vi "Write Range UI.vi"(8 "error in (no error)":errorcluster, 9 "Reader Time":dbl[unit], 10 "Set UI to input? (F)":bool, 11 "Double Scanner in":refnum<class "Double Scanner.lvclass">) -> (0 "error out":errorcluster, 3 "Double Scanner out":refnum<class "Double Scanner.lvclass">)   [LabVIEW 2012, in "Double Scanner.lvclass"]
doc: "A Setup UI method for the superclass \"Range\" of scanner."
uses:
  Double Scanner.lvclass
  Scanner/Scanner.lvclass
  Scanner/Range.ctl
panel:
  out "# Points":u32
  out "Time Estimate":string
  in  "Tab Control":enum32{"Range 1", "Range 2"}(tab)
  in  "First 1":dbl
  in  "Last 1":dbl
  in  "Step Size 1":dbl=1.0 min=0.0
  in  "Return to 1":dbl
  in  "Return to...? 1":bool
  in  "First 2":dbl
  in  "Last 2":dbl
  in  "Step Size 2":dbl=1.0 min=0.0
  in  "Return to 2":dbl
  in  "Return to...? 2":bool
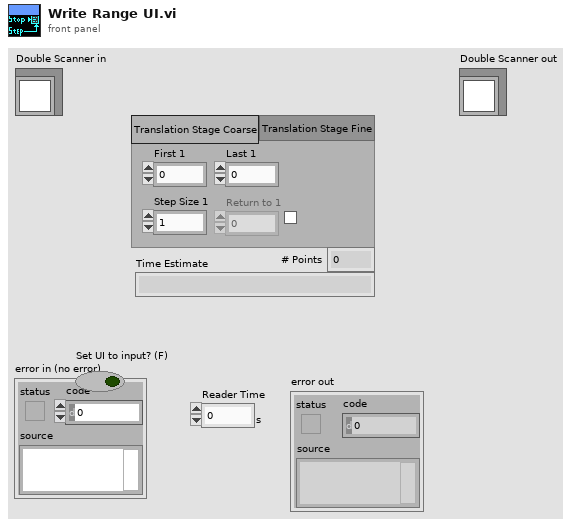
[diagram p1: front panel]
types:
  T1 = typedef "Scanner.lvclass/Range.ctl" = cluster{"xi":dbl, "xf":dbl, "dx":dbl, "Return to...?":bool, "Return to":dbl}
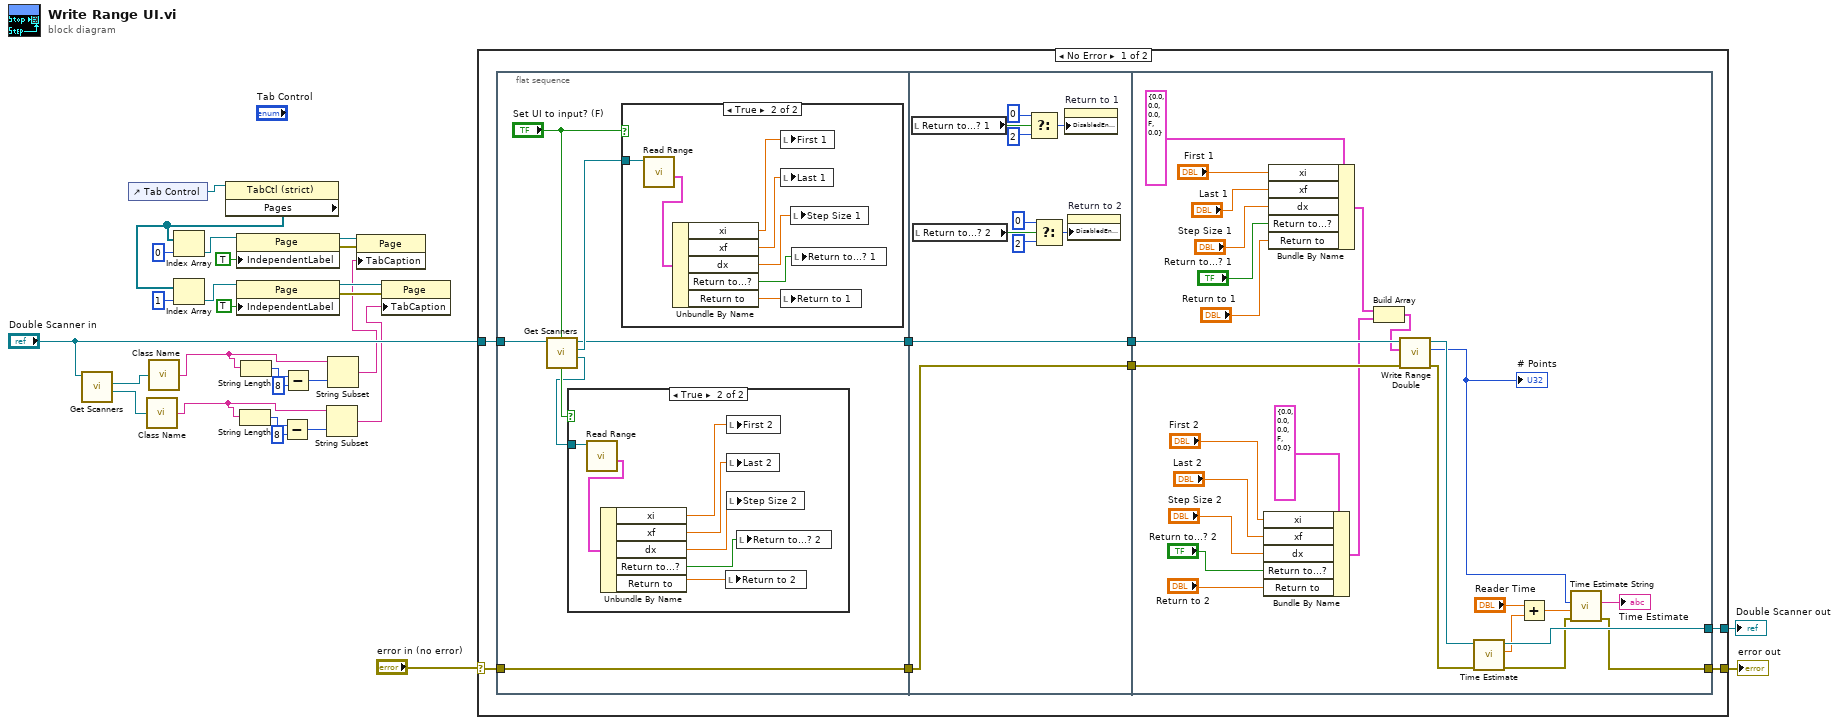
[diagram p0: block diagram]
diagram:
  n1 = call-dynamic "Get Scanners.vi"("Double Scanner in"="Double Scanner in") -> ("Scanner 2 out"=w23:refnum<class "Scanner.lvclass">, "Scanner 1 out"=w24:refnum<class "Scanner.lvclass">)  [unwired: 7 in, 2 out]
  n2 = control-ref of="Tab Control"() -> (w22:refnum<vi>)
  n3 = call "Class Name.vi"("LabVIEW Object"=w23) -> ("Classname"=w1:string)
  n4 = call "Class Name.vi"("LabVIEW Object"=w24) -> ("Classname"=w6:string)
  n5 = property class="TabCtl (strict)"(reference=w22) -> ("Pages"=w20:refnum<vi>[])  [unwired: 1 in, 2 out]
  n6 = Index Array(array=w20, index=0) -> (element=w17:refnum<vi>)
  n7 = Index Array(array=w20, index=1) -> (element=w18:refnum<vi>)
  n8 = property class="Page"(reference=w17, "IndependentLabel"=TRUE ("Independent Label")) -> (reference out=w13:refnum<vi>, error out=w12:errorcluster)  [unwired: 1 in]
  n9 = property class="Page"(reference=w18, "IndependentLabel"=TRUE ("Independent Label")) -> (reference out=w14:refnum<vi>, error out=w11:errorcluster)  [unwired: 1 in]
  n10 = String Length(string=w1) -> (length=w5:i32)
  n11 = String Length(string=w6) -> (length=w10:i32)
  n12 = Subtract(x=w5, y=8) -> (x-y=w3:i32)
  n13 = Subtract(x=w10, y=8) -> (x-y=w7:i32)
  n14 = String Subset(string=w1, length (rest)=w3) -> (substring=w2:string)  [unwired: 1 in]
  n15 = String Subset(string=w6, length (rest)=w7) -> (substring=w8:string)  [unwired: 1 in]
  n16 = property class="Page"(reference=w13, error in=w12, "TabCaption"=w8) -> ()  [unwired: 2 out]
  n17 = property class="Page"(reference=w14, error in=w11, "TabCaption"=w2) -> ()  [unwired: 2 out]
  n18 = case shown="No Error" "error in (no error)" {
    selector: "error in (no error)" -> [w35 w95]
    tunnel: [w33 w95] -> w27
    tunnel: [w34 w94] -> w28
    tunnel: "Double Scanner in" -> [w36 w94]
    frame No Error {
      n19 = flat-sequence {
        tunnel: w35 -> [w42]
        tunnel: w36 -> [w40]
        tunnel: [w37] -> w32
        tunnel: [w42] -> w30
        tunnel: w32 -> [w66]
        tunnel: [w66] -> w31
        tunnel: w30 -> [w57]
        tunnel: [w57] -> w29
        tunnel: [w76] -> w34
        tunnel: [w67] -> w33
        tunnel: w31 -> [w81]
        tunnel: w29 -> [w80]
        frame #0 {
          n20 = call-dynamic "Get Scanners.vi"("Double Scanner in"=w40) -> ("Scanner 2 out"=w39:refnum<class "Scanner.lvclass">, "Scanner 1 out"=w38:refnum<class "Scanner.lvclass">, "Double Scanner out"=w37:refnum<class "Double Scanner.lvclass">)  [unwired: 7 in, 1 out]
          n21 = case shown="True" "Set UI to input? (F)" {
            tunnel: w39 -> [_ w49]
            frame False {
            }
            frame True {
              n22 = call-dynamic "Read Range.vi"("Scanner.lvclass in"=w49) -> ("Range"=w48:T1)  [unwired: 5 in, 5 out]
              n23 = Unbundle By Name(w48) -> ("xi"=w47:dbl, "xf"=w46:dbl, "dx"=w45:dbl, "Return to...?"=w44:bool, "Return to"=w43:dbl)
              n24 = local write "Return to 2"(w43) -> ()
              n25 = local write "First 2"(w47) -> ()
              n26 = local write "Last 2"(w46) -> ()
              n27 = local write "Step Size 2"(w45) -> ()
              n28 = local write "Return to...? 2"(w44) -> ()
            }
          }
          n29 = case shown="True" "Set UI to input? (F)" {
            tunnel: w38 -> [_ w56]
            frame False {
            }
            frame True {
              n30 = call-dynamic "Read Range.vi"("Scanner.lvclass in"=w56) -> ("Range"=w55:T1)  [unwired: 5 in, 5 out]
              n31 = Unbundle By Name(w55) -> ("xi"=w54:dbl, "xf"=w53:dbl, "dx"=w52:dbl, "Return to...?"=w51:bool, "Return to"=w50:dbl)
              n32 = local write "First 1"(w54) -> ()
              n33 = local write "Last 1"(w53) -> ()
              n34 = local write "Return to 1"(w50) -> ()
              n35 = local write "Step Size 1"(w52) -> ()
              n36 = local write "Return to...? 1"(w51) -> ()
            }
          }
        }
        frame #1 {
          n37 = local read "Return to...? 1"() -> (w64:bool)
          n38 = local read "Return to...? 2"() -> (w58:bool)
          n39 = Select(t=0, s=w64, f=2) -> (s? t:f=w65:i32)
          n40 = Select(t=0, s=w58, f=2) -> (s? t:f=w59:i32)
          n41 = property on="Return to 1" class="DigNum (strict)"("DisabledEnum"=w65) -> ()  [unwired: 2 in, 2 out]
          n42 = property on="Return to 2" class="DigNum (strict)"("DisabledEnum"=w59) -> ()  [unwired: 2 in, 2 out]
        }
        frame #2 {
          n43 = Bundle By Name(cluster=T1 {"xi"=0.0, "xf"=0.0, "dx"=0.0, "Return to...?"=FALSE, "Return to"=0.0} ("Range"), "xi"="First 2", "xf"="Last 2", "dx"="Step Size 2", "Return to...?"="Return to...? 2", "Return to"="Return to 2") -> (w78:T1)
          n44 = Bundle By Name(cluster=T1 {"xi"=0.0, "xf"=0.0, "dx"=0.0, "Return to...?"=FALSE, "Return to"=0.0} ("Range"), "xi"="First 1", "xf"="Last 1", "dx"="Step Size 1", "Return to...?"="Return to...? 1", "Return to"="Return to 1") -> (w77:T1)
          n45 = Build Array(w77, w78) -> (w79:T1[])
          n46 = call-dynamic "Write Range Double.vi"("error in (no error)"=w80, "Range Array"=w79, "Double Scanner in"=w81) -> ("error out"=w74:errorcluster, "# Points"=w70:u32, "Double Scanner out"=w75:refnum<class "Double Scanner.lvclass">)  [unwired: 6 in]
          "# Points" <- w70
          n47 = call-dynamic "Time Estimate.vi"("error in (no error)"=w74, "Double Scanner.lvclass"=w75) -> ("error out"=w68:errorcluster, "time"=w72:dbl[unit], "Double Scanner.lvclass out"=w76:refnum<class "Double Scanner.lvclass">)  [unwired: 2 in, 5 out]
          n48 = Add(x="Reader Time", y=w72) -> (x+y=w71:dbl[unit])
          n49 = call "Time Estimate String.vi"("error in (no error)"=w68, "Time"=w71, "Steps"=w70) -> ("error out"=w67:errorcluster, "Time Estimate String"=→"Time Estimate":string)  [unwired: 7 in]
        }
      }
    }
    frame Error {
    }
  }
  "error out" <- w27
  "Double Scanner out" <- w28
